vi "Spaced Camel Case Converter.vi"(4 "Input string":string) -> (1 "Output string":string)   [LabVIEW 2025, in "Name Formatter.lvlib"]
doc: "Description:\nTransforms a text with words separated by spaces into <b>#SpacedCamelCase</b>. Each word starts with an uppercase letter, and spaces are preserved.\n\nExample:\nInput -> hello cruel cruel\nOutput -> helloCruelWorld\n\nRequirements:\nThe input must contain spaces. Without spaces, this conversion cannot be applied."
uses:
  Name Formatter.lvlib
panel:
  # "text with spaces"
  # "Spaced Camel Case"
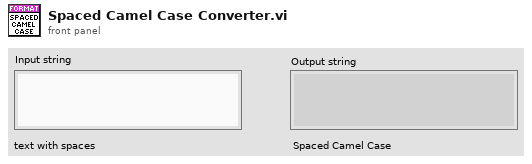
[diagram p1: front panel]
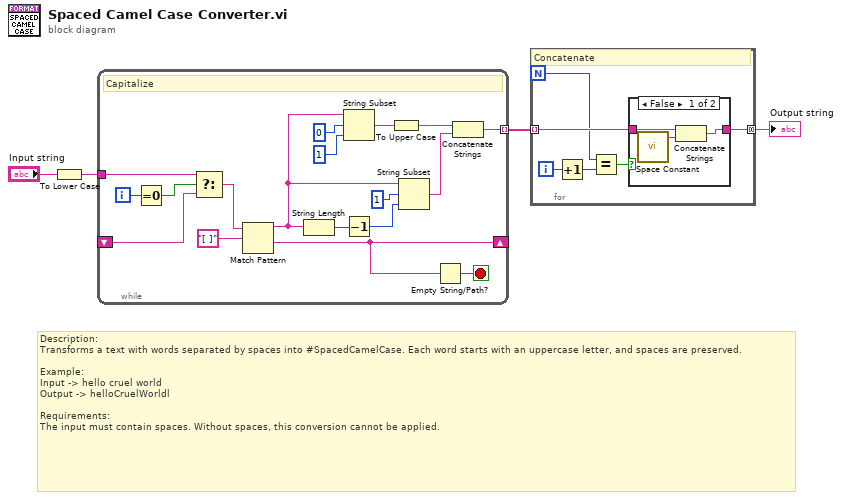
[diagram p0: block diagram]
diagram:
  # "Description:\nTransforms a text with words separated by spaces into #SpacedCamelCase. Each word starts with an uppercase letter, and spaces are preserved.\n\nExample:\nInput -> hello cruel world\nOutput -> helloCruelWorldl\n\nRequirements:\nThe input must contain spaces. Without spaces, this conversion cannot be applied."
  n1 = To Lower Case(string="Input string") -> (all lower case string=w1:string)
  n2 = while {
    tunnel: w1 -> [w21]
    tunnel: [w8] -> w3 mode=indexing
    shift-right: [w18] -> _
    shift-left: _ -> [w19]
    i -> [w6]
    stop <- w17 stop-if-true
    # "Capitalize"
    n3 = Equal To 0?(x=w6) -> (x = 0?=w5:bool)
    n4 = Select(t=w21, s=w5, f=w19) -> (s? t:f=w20:string)
    n5 = Match Pattern(string=w20, regular expression="[ ]") -> (before substring=w7:string, after substring=w18:string)  [unwired: 1 in, 2 out]
    n6 = String Length(string=w7) -> (length=w12:i32)
    n7 = String Subset(string=w7, offset (0)=0, length (rest)=1 ("length (rest)")) -> (substring=w15:string)
    n8 = Decrement(x=w12) -> (x-1=w11:i32)
    n9 = To Upper Case(1:w15) -> (0:w10:string)
    n10 = String Subset(string=w7, offset (0)=1, length (rest)=w11) -> (substring=w9:string)
    n11 = Empty String/Path?(string/path=w18) -> (empty?=w17:bool)
    n12 = Concatenate Strings(w10, w9) -> (w8:string)
  }
  n13 = for {
    N -> [w25]
    tunnel: w3 -> [w28] mode=indexing
    tunnel: [w27] -> w2 mode=concatenating
    i -> [w26]
    # "Concatenate"
    n14 = Increment(x=w26) -> (x+1=w24:i32)
    n15 = Equal?(x=w25, y=w24) -> (x = y?=w23:bool)
    n16 = case shown="False" w23 {
      tunnel: w28 -> [w31 w32]
      tunnel: [w29 w32] -> w27
      frame False {
        n17 = call <vilib>:"Space Constant.vi"() -> ("String"=w30:string)
        n18 = Concatenate Strings(w31, w30) -> (w29:string)
      }
      frame True {
      }
    }
  }
  "Output string" <- w2
